vi "Set Delay.vi"(8 "error in (no error)":errorcluster, 9 "Rate (ps/s)":dbl, 10 "Delay (ps)":dbl, 11 "Instrument.DelayLine in":refnum<class "Instrument.DelayLine.lvclass">) -> (0 "error out":errorcluster, 3 "Instrument.DelayLine out":refnum<class "Instrument.DelayLine.lvclass">)   [LabVIEW 2019, in "Instrument.DelayLine.lvclass"]
uses:
  Instrument.DelayLine.lvclass
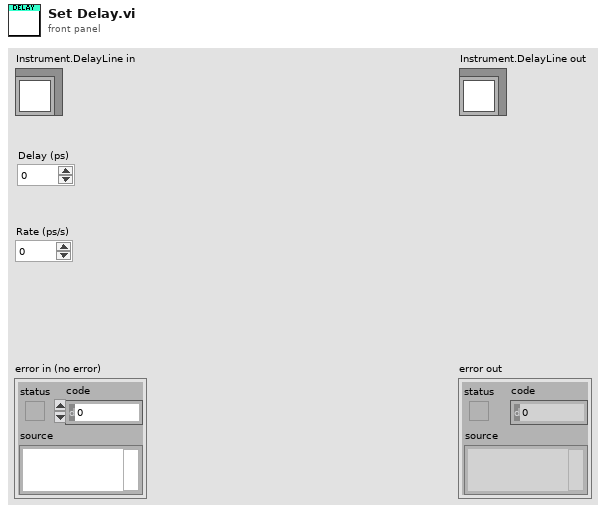
[diagram p1: front panel]
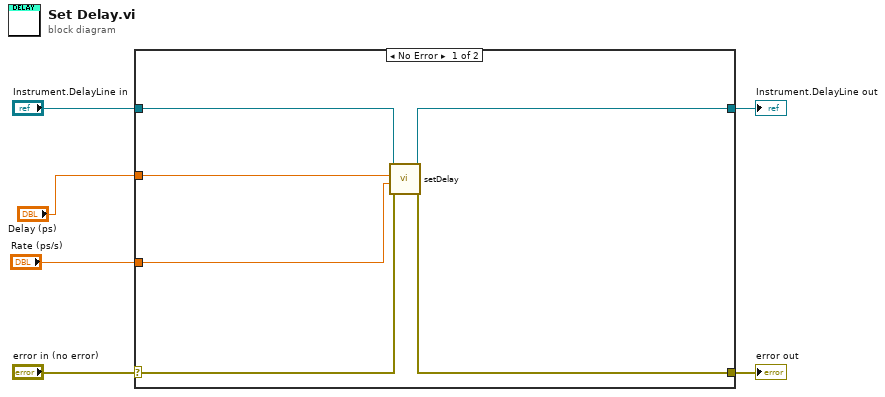
[diagram p0: block diagram]
diagram:
  n1 = case shown="No Error" "error in (no error)" {
    selector: "error in (no error)" -> [w10 w14]
    tunnel: [w9 w14] -> w5
    tunnel: [w12 w13] -> w3
    tunnel: "Instrument.DelayLine in" -> [w11 w13]
    tunnel: "Rate (ps/s)" -> [w8 _]
    tunnel: "Delay (ps)" -> [w7 _]
    frame No Error {
      n2 = call-dynamic "setDelay.vi"("error in (no error)"=w10, "Rate (ps/s)"=w8, "Delay (ps)"=w7, "Instrument.Delay in"=w11) -> ("error out"=w9:errorcluster, "Instrument.Delay out"=w12:refnum<class "Instrument.DelayLine.lvclass">)  [unwired: 6 in]
    }
    frame Error {
    }
  }
  "error out" <- w5
  "Instrument.DelayLine out" <- w3
